vi "Write ref.vi"(8 "error in (no error)":errorcluster, 10 "ref":refnum<k24>, 11 "Query Result in":refnum<class "DapperResult.lvclass">) -> (0 "error out":errorcluster, 3 "Query Result out":refnum<class "DapperResult.lvclass">)   [LabVIEW 2020, in "ORM_Dapper.lvlib" / "DapperResult.lvclass"]
uses:
  DapperResult.lvclass
  DapperResult.lvclass/DapperResult.ctl
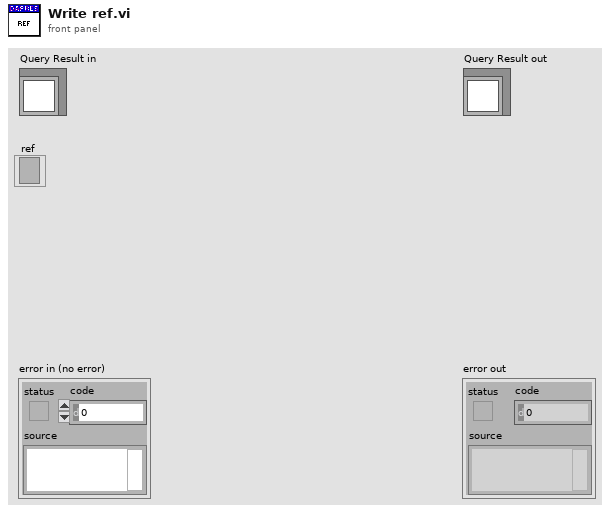
[diagram p1: front panel]
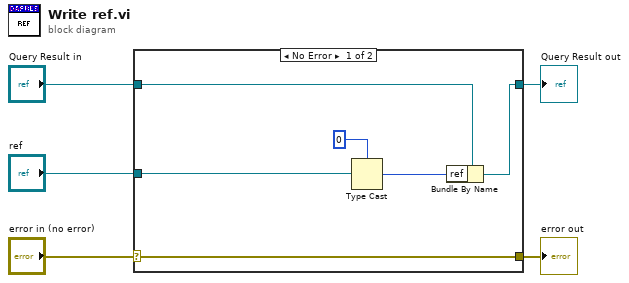
[diagram p0: block diagram]
diagram:
  n1 = case shown="No Error" "error in (no error)" {
    selector: "error in (no error)" -> [w11 w12]
    tunnel: [w11 w12] -> w4
    tunnel: [w9 w13] -> w2
    tunnel: "Query Result in" -> [w10 w13]
    tunnel: "ref" -> [w8 _]
    frame No Error {
      n2 = Type Cast(type=u64 0 ("ref"), x=w8) -> (*(type *) &x=w6:u64)
      n3 = Bundle By Name(cluster=w10, "ref"=w6) -> (w9:refnum<class "DapperResult.lvclass">)
    }
    frame Error {
    }
  }
  "error out" <- w4
  "Query Result out" <- w2
